vi "ep_EN50160 Basic Statistical Evaluation (3D).vi"(0 "data":dbl[][][](array[numeric]), 1 "evaluated data":enum16{"all data", "data without flag"}(ring), 5 "data flags":bool[][](array[boolean]), 7 "EN50160 limits":T2(array[cluster]), 11 "error in (no error)":errorcluster) -> (4 "EN50160 results":T1(array[cluster]), 10 "passed?":bool, 15 "error out":errorcluster)   [LabVIEW 2011, in "NI_EP_Power Quality.lvlib"]
uses:
  <vilib>/addons/Electrical Power/PQ/NI_EP_Power Quality.lvlib
  <vilib>/addons/Electrical Power/PQ/Utility/subVIs/ep_EN50160 Basic Statistical Evaluation (2D).vi
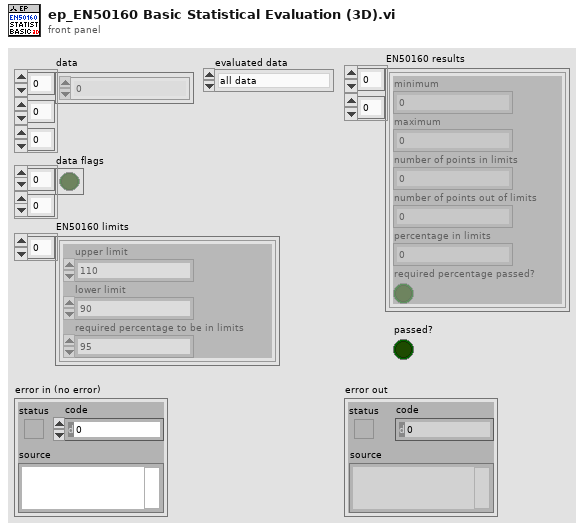
[diagram p1: front panel]
types:
  T1 = cluster{"minimum":dbl, "maximum":dbl, "number of points in limits":u32, "number of points out of limits":u32, "percentage in limits":dbl, "required percentage passed?":bool}[][]
  T2 = cluster{"upper limit":dbl, "lower limit":dbl, "required percentage to be in limits":dbl}[]
  T3 = cluster{"minimum":dbl, "maximum":dbl, "number of points in limits":u32, "number of points out of limits":u32, "percentage in limits":dbl, "required percentage passed?":bool}[]
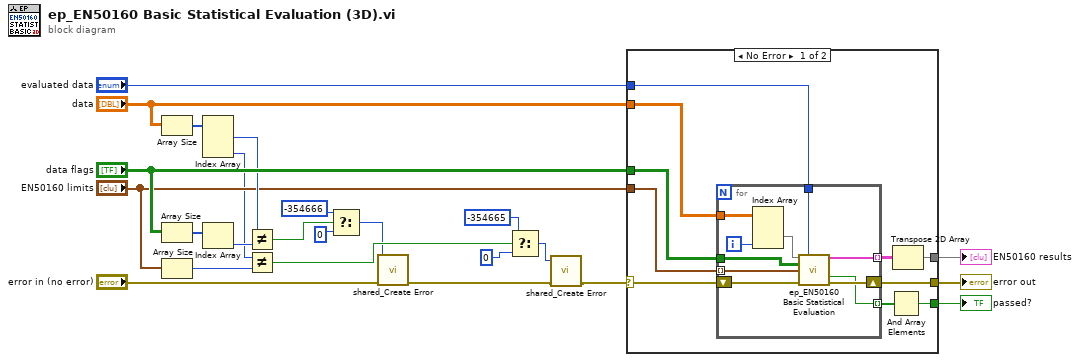
[diagram p0: block diagram]
diagram:
  n1 = Array Size(array="data") -> (size(s)=w19:i32[])
  n2 = Array Size(array="data flags") -> (size(s)=w18:i32[])
  n3 = Array Size(array="EN50160 limits") -> (size(s)=w13:i32)
  n4 = Index Array(array=w19) -> (element #1=w15:i32, element #3=w10:i32)  [unwired: 3 in, 1 out]
  n5 = Index Array(array=w18) -> (element=w17:i32)  [unwired: 1 in]
  n6 = Not Equal?(x=w15, y=w17) -> (x != y?=w16:bool)
  n7 = Not Equal?(x=w10, y=w13) -> (x != y?=w12:bool)
  n8 = Select(t=-354666, s=w16, f=0 ("error code (0)")) -> (s? t:f=w6:i32)
  n9 = call <vilib>:"shared_Create Error.vi"("error in (no error)"="error in (no error)", "error code (0)"=w6) -> ("error out"=w4:errorcluster)  [unwired: 9 in]
  n10 = Select(t=-354665 ("error code (0)"), s=w12, f=0 ("error code (0)")) -> (s? t:f=w2:i32)
  n11 = call <vilib>:"shared_Create Error.vi"("error in (no error)"=w4, "error code (0)"=w2) -> ("error out"=w3:errorcluster)  [unwired: 9 in]
  n12 = case shown="No Error" w3 {
    selector: w3 -> [w30 w45]
    tunnel: "evaluated data" -> [w31 _]
    tunnel: "data" -> [w26 _]
    tunnel: "data flags" -> [w34 _]
    tunnel: [w29 w45] -> w23
    tunnel: [w25 _] -> w22
    tunnel: "EN50160 limits" -> [w33 _]
    tunnel: [w27 _] -> w11
    frame No Error {
      n13 = for {
        tunnel: w26 -> [w37]
        tunnel: w34 -> [w44]
        tunnel: w33 -> [w43] mode=indexing
        tunnel: [w42] -> w32 mode=indexing
        tunnel: w31 -> [w41]
        shift-right: [w39] -> w29
        shift-left: w30 -> [w40]
        tunnel: [w38] -> w28 mode=indexing
        i -> [w36]
        n14 = Index Array(array=w37, index (dim 2)=w36) -> (element=w35:dbl[][])  [unwired: 2 in]
        n15 = call-poly <vilib>:"ep_EN50160 Basic Statistical Evaluation.vi"("data"=w35, "evaluated data"=w41, "data flags"=w44, "EN50160 limits"=w43, "error in (no error)"=w40) -> ("EN50160 results"=w42:T3, "passed?"=w38:bool, "error out"=w39:errorcluster)  [unwired: 8 in]
      }
      n16 = And Array Elements(Boolean array=w28) -> (logical AND=w27:bool)
      n17 = Transpose 2D Array(2D array=w32) -> (transposed array=w25:T1)
    }
    frame Error {
    }
  }
  "EN50160 results" <- w22
  "error out" <- w23
  "passed?" <- w11
